vi "Launcher.vi"() -> ()   [LabVIEW 2018, in "MonSys_Client_Actor.lvlib" / "MonSys_Client_Actor.lvclass"]
uses:
  MonSys_Client_Actor.lvclass
  <vilib>/ActorFramework/Message Enqueuer/Message Enqueuer.lvclass
  C:/Program Files (x86)/National Instruments/LabVIEW 2018/vi.lib/ActorFramework/Actor/Actor.lvclass
  <vilib>/ActorFramework/Message Enqueuer/Message Enqueuer.lvclass/Message Enqueuer.ctl
  <vilib>/ActorFramework/Message Enqueuer/Enqueue.vi
  <vilib>/ActorFramework/Stop Msg/Stop Msg.lvclass
  C:/Program Files (x86)/National Instruments/LabVIEW 2018/vi.lib/ActorFramework/Message/Message.lvclass
  <vilib>/ActorFramework/Message Priority Queue/Priority Enqueue.vi
  <vilib>/ActorFramework/Actor/Actor.lvclass
panel:
  in  "Stop":bool
  in  "port":string="8001"
  in  "IP_Address":string="127.0.0.1"
  in  "launch_new_actor":bool
  # "Monitoring System"
  # "enter IP address and port from your target system"
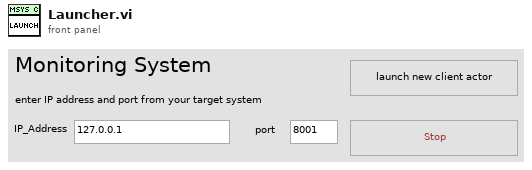
[diagram p1: front panel]
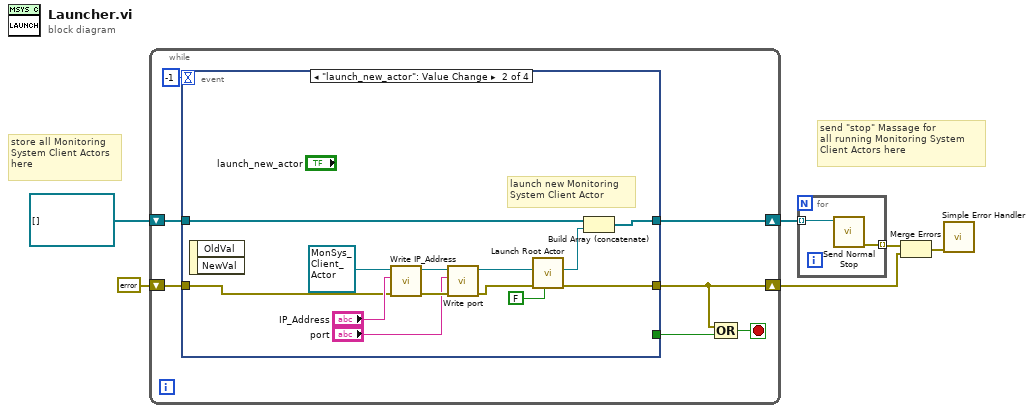
[diagram p0: block diagram]
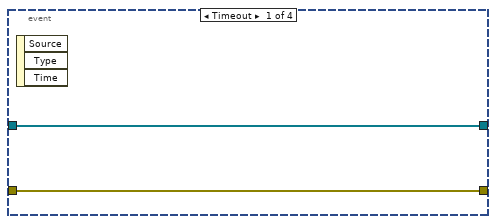
[diagram p2: hidden frame]
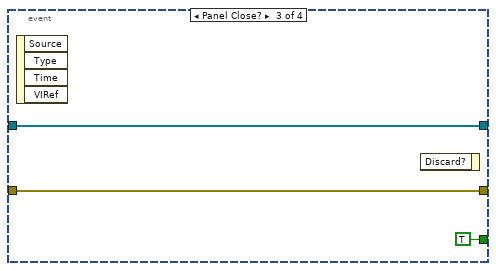
[diagram p3: hidden frame]
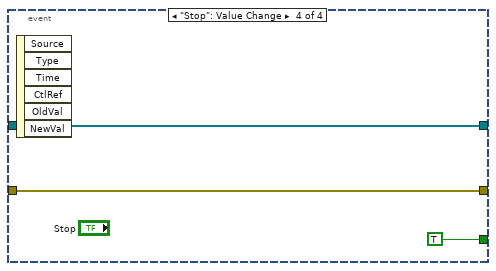
[diagram p4: hidden frame]
diagram:
  # "send \"stop\" Massage for \nall running Monitoring System \nClient Actors here"
  # "store all Monitoring\nSystem Client Actors\nhere"
  n1 = while {
    shift-right: [w10] -> w2
    shift-left: errorcluster {"status"=FALSE, "code"=0, "source"=""} ("error out") -> [w12]
    shift-right: [w8] -> w4
    shift-left: refnum<class "Message Enqueuer.lvclass">[] [] -> [w7]
    stop <- w11 stop-if-true
    n2 = event shown="[1] \"launch_new_actor\": Value Change" {
      selector: _ -> [_ _ _ _]
      dyn-events: _ -> [_ _ _ _]
      timeout: -1 -> [_ _ _ _]
      tunnel: [w15 w20 w30 w33] -> w10
      tunnel: w12 -> [w15 w19 w30 w33]
      tunnel: [_ _ TRUE ("Stop") TRUE ("Stop")] -> w9
      tunnel: [w14 w17 w29 w32] -> w8
      tunnel: w7 -> [w14 w16 w29 w32]
      event Timeout {
        n3 = event-data() -> ()  [unwired: 1 in, 3 out]
      }
      event "launch_new_actor": Value Change {
        # "launch new Monitoring\nSystem Client Actor"
        n4 = event-data() -> ()  [unwired: 1 in, 2 out]
        n5 = call-dynamic "Write IP_Address.vi"("error in (no error)"=w19, "IP_Address"="IP_Address", "MonSys_Client_Actor in"=refnum<class "MonSys_Client_Actor.lvclass"> refnum ("MonSys_Client_Actor.lvlib:MonSys_Client_Actor.lvclass")) -> ("error out"=w26:errorcluster, "MonSys_Client_Actor out"=w28:refnum<class "MonSys_Client_Actor.lvclass">)  [unwired: 7 in]
        n6 = call-dynamic "Write port.vi"("error in (no error)"=w26, "port"="port", "MonSys_Client_Actor in"=w28) -> ("error out"=w25:errorcluster, "MonSys_Client_Actor out"=w27:refnum<class "MonSys_Client_Actor.lvclass">)  [unwired: 7 in]
        n7 = call <vilib>:"Launch Root Actor.vi"("Open Actor Core front panel? (F)"=FALSE, "error in (no error)"=w25, "Actor"=w27) -> ("error out"=w20:errorcluster, "Actor's Enqueuer"=w18:refnum<class "Message Enqueuer.lvclass">)  [unwired: 7 in]
        n8 = Build Array (concatenate)(w16, w18) -> (w17:refnum<class "Message Enqueuer.lvclass">[])
      }
      event Panel Close? {
        n9 = event-data() -> ()  [unwired: 1 in, 4 out]
        n10 = event-data() -> ()  [unwired: 2 in, 1 out]
      }
      event "Stop": Value Change {
        n11 = event-data() -> ()  [unwired: 1 in, 6 out]
      }
    }
    n12 = Compound Arithmetic op=OR(w10, w9) -> (w11:bool)
  }
  n13 = for {
    tunnel: w4 -> [w36] mode=indexing
    tunnel: [w35] -> w3 mode=indexing
    n14 = call <vilib>:"Send Normal Stop.vi"("Message Enqueuer"=w36) -> ("error out"=w35:errorcluster)  [unwired: 10 in]
  }
  n15 = Merge Errors(w3, w2) -> (w1:errorcluster)
  n16 = call <vilib>:"Simple Error Handler.vi"("error in (no error)"=w1) -> ()  [unwired: 4 in, 5 out]
